vi "Read Event Type.vi"(8 "error in (no error)":errorcluster, 11 "VI in":refnum<class "VI.lvclass">) -> (0 "error out":errorcluster, 2 "Event Type (New)":T1, 3 "VI out":refnum<class "VI.lvclass">)   [LabVIEW 2019]
uses:
  VI.lvclass
  <vilib>/Delacor/Delacor QMH/Libraries/_Scripting Support/Event Type (New)--enum.ctl
  VI.lvclass/VI.ctl
  <vilib>/Delacor/Delacor QMH/Libraries/_Scripting Support/dqmh_lib_DQMH Scripting Support.lvlib
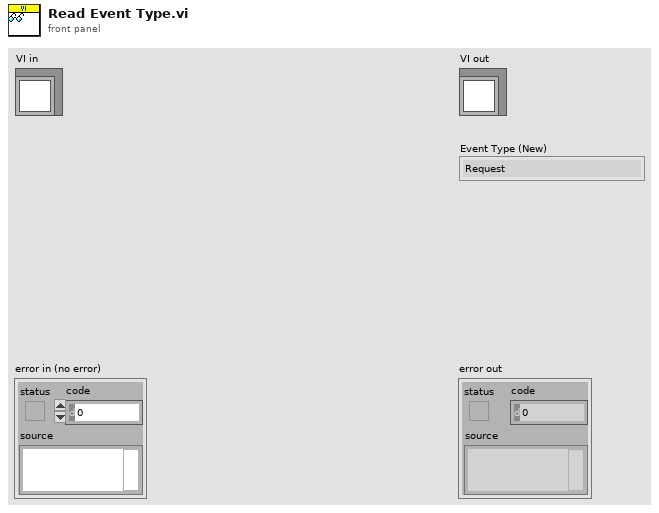
[diagram p1: front panel]
types:
  T1 = typedef "dqmh_lib_DQMH Scripting Support.lvlib/Event Type (New)--enum.ctl" = enum16{"Request", "Broadcast", "Request and Wait for Reply", "Round Trip"}
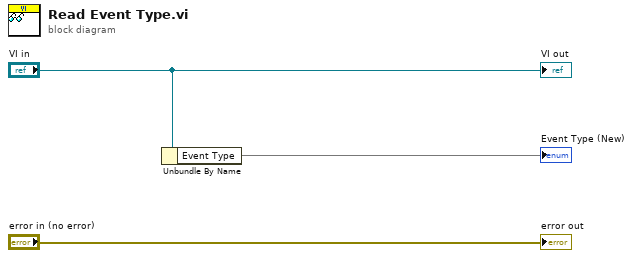
[diagram p0: block diagram]
diagram:
  n1 = Unbundle By Name("VI in") -> ("Event Type"=→"Event Type (New)")
  "error out" <- "error in (no error)"
  "VI out" <- "VI in"
